vi "dB, degrees to Z.vi"(1 "Magnitude (dB)":dbl[](array[numeric]), 2 "Phase (degrees)":dbl[](array[numeric])) -> (6 "Z":cdb[](array[numeric]))   [LabVIEW 2020]
uses:
  4aaeeaf8-f178-4447-89ad-0513212895d8.vi
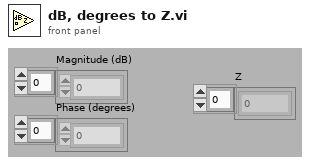
[diagram p1: front panel]
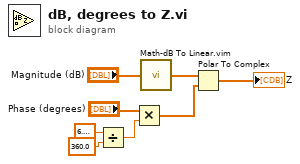
[diagram p0: block diagram]
diagram:
  n1 = Divide(x=6.283185307179586, y=360.0) -> (x/y=w3:dbl)
  n2 = Multiply(x="Phase (degrees)", y=w3) -> (x*y=w5:dbl[])
  n3 = call "Math-dB To Linear.vim"("dB"="Magnitude (dB)") -> ("linear"=w7:dbl[])
  n4 = Polar To Complex(1:w5, 2:w7) -> (0:→"Z":cdb[])
